vi "set severity.vi"(10 "severity":T1, 11 "exception in":T2 {"code" format="%.0x"}) -> (3 "exception out":T2 {"code" format="%.0x"})   [LabVIEW 2013, in "exception.lvlib"]
uses:
  exception.lvlib
  exception.ctl
  severity.ctl
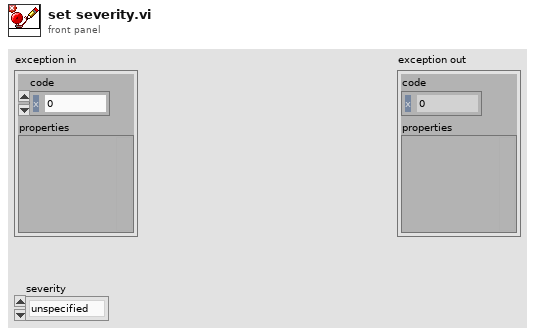
[diagram p1: front panel]
types:
  T1 = typedef "exception.lvlib/severity.ctl" = enum8{"unspecified", "operation failed", "data corruption", "system corruption", "critical unknown state"}
  T2 = typedef "exception.lvlib/exception.ctl" = cluster{"code":i32, "properties":variant}
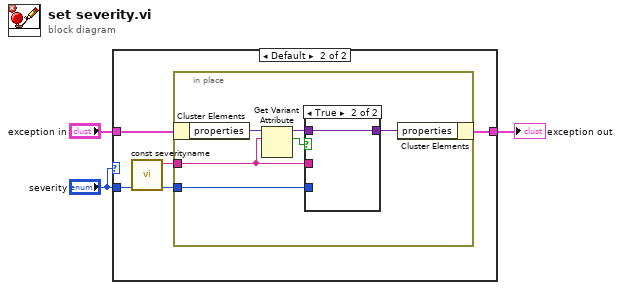
[diagram p0: block diagram]
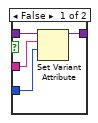
[diagram p3: hidden frame]
diagram:
  n1 = case shown="Default" "severity" {
    tunnel: "exception in" -> [w4 w8]
    tunnel: [w4 w7] -> w2
    tunnel: "severity" -> [_ w6]
    frame "unspecified" {
    }
    frame Default {
      n2 = call "const severityname.vi"() -> ("label"=w5:string)  [unwired: 11 in]
      n3 = in-place {
        in-place-border: w5 -> [w9]
        in-place-border: w6 -> [w13]
        n4 = in-place-cluster #1(w8) -> ("properties"=w12:variant)
        n5 = Get Variant Attribute(Variant=w12, name=w9) -> (duplicate Variant=w11:variant, found=w10:bool)  [unwired: 2 in, 2 out]
        n6 = case shown="True" w10 {
          tunnel: w11 -> [w18 w19]
          tunnel: [w17 w19] -> w14
          tunnel: w9 -> [w16 _]
          tunnel: w13 -> [w15 _]
          frame False {
            n7 = Set Variant Attribute(Variant=w18, name=w16, value=w15) -> (Variant out=w17:variant)  [unwired: 1 in, 2 out]
          }
          frame True {
          }
        }
        n8 = in-place-cluster #1("properties"=w14) -> (w7:T2)
      }
    }
  }
  "exception out" <- w2
